vi "ReadSnapshot.vi"(0 "Buffers in":T1={"Channels"=[], "PosttriggerBuffer"=refnum, "PretriggerBuffer"=refnum, "BlockSizePerChannel"=0, " logging semaphore"=refnum, "Log refnum"=refnum, "snapshotBuffer"=refnum, "logDirectory"=path "", "logPrefix"="", "decimation factor"=1, "max files"=0, "SampleRate"=0.0}, 5 "sizeOfBlock":i32, 11 "error in (no error)":errorcluster) -> (4 "Buffers out":T1={"Channels"=[], "PosttriggerBuffer"=refnum, "PretriggerBuffer"=refnum, "BlockSizePerChannel"=0, " logging semaphore"=refnum, "Log refnum"=refnum, "snapshotBuffer"=refnum, "logDirectory"=path "", "logPrefix"="", "decimation factor"=1, "max files"=0, "SampleRate"=0.0}, 6 "snapshot":sgl[][](array[numeric]), 15 "error out":errorcluster)   [LabVIEW 2017, in "BufferLogging.lvlib"]
uses:
  BufferLogging.lvlib
  Buffers.ctl
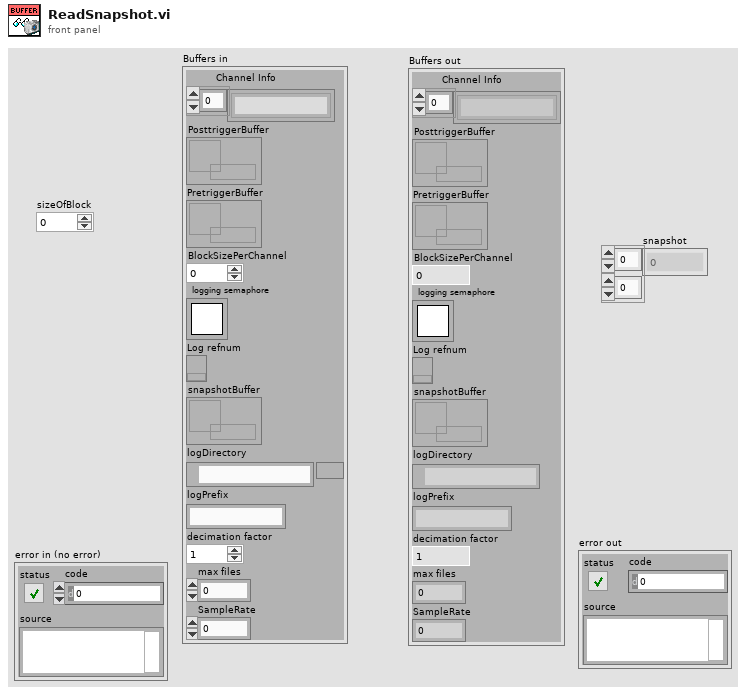
[diagram p1: front panel]
types:
  T1 = typedef "BufferLogging.lvlib/Buffers.ctl" = cluster{"Channels":string[], "PosttriggerBuffer":refnum<queue>, "PretriggerBuffer":refnum<queue>, "BlockSizePerChannel":i32, " logging semaphore":T2, "Log refnum":refnum<k34>, "snapshotBuffer":refnum<data-value>, "logDirectory":path, "logPrefix":string, "decimation factor":i32, "max files":i32, "SampleRate":dbl}
  T2 = typedef "Semaphore RefNum" = refnum<k1>
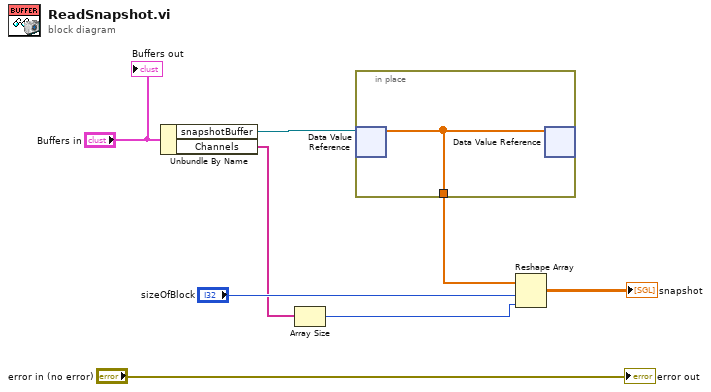
[diagram p0: block diagram]
diagram:
  n1 = Unbundle By Name("Buffers in") -> ("snapshotBuffer"=w7:refnum<data-value>, "Channels"=w2:string[])
  n2 = Array Size(array=w2) -> (size(s)=w1:i32)
  n3 = in-place {
    in-place-border: [w9] -> w6
    n4 = in-place-dvr #1(w7) -> (w9:sgl[])  [unwired: 1 out]
    n5 = in-place-dvr #1(w9) -> ()  [unwired: 2 out]
  }
  n6 = Reshape Array(w6, "sizeOfBlock", w1) -> (→"snapshot":sgl[][])
  "error out" <- "error in (no error)"
  "Buffers out" <- "Buffers in"
